vi "Create Song.vi"(0 "Name":string, 5 "Duration (s)":T1 format="%<%M:%S>T", 7 "Artist":string, 9 "Album":string, 11 "error in (no error)":errorcluster) -> (4 "Song out":refnum<class "Song.lvclass">, 15 "error out":errorcluster)   [LabVIEW 2015, in "Song.lvclass"]
uses:
  Song.lvclass
  Song Duration.ctl
  Song.lvclass/Song.ctl
  Write Duration (s).vi
  Write Artist.vi
  Write Album.vi
  MusicElement.lvclass
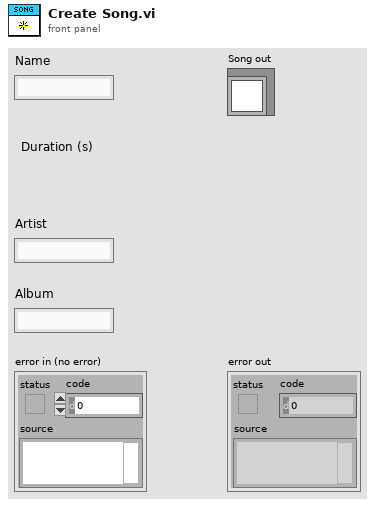
[diagram p1: front panel]
types:
  T1 = typedef "Song.lvclass/Song Duration.ctl" = timestamp
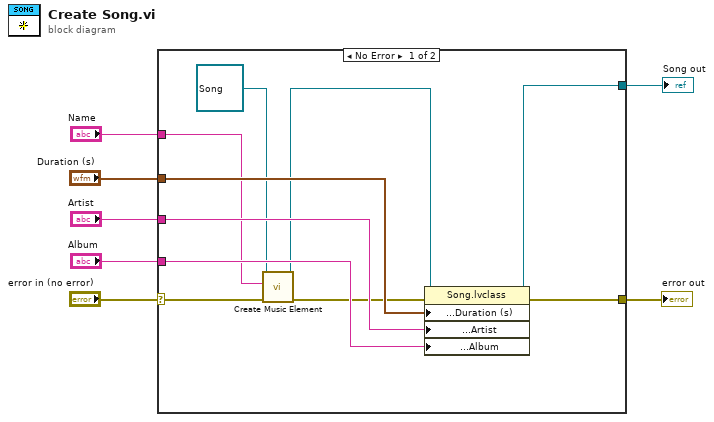
[diagram p0: block diagram]
diagram:
  n1 = case shown="No Error" "error in (no error)" {
    selector: "error in (no error)" -> [w12 w18]
    tunnel: [w16 w18] -> w6
    tunnel: "Name" -> [w8 _]
    tunnel: [w17 _] -> w4
    tunnel: "Artist" -> [w15 _]
    tunnel: "Album" -> [w14 _]
    tunnel: "Duration (s)" -> [w13 _]
    frame No Error {
      n2 = call "Create Music Element.vi"("error in (no error)"=w12, "Name"=w8, "MusicElement in"=refnum<class "Song.lvclass"> refnum ("Song out")) -> ("error out"=w9:errorcluster, "MusicElement out"=w10:refnum<class "Song.lvclass">)  [unwired: 7 in]
      n3 = property class="Song.lvclass"(reference=w10, error in=w9, "API:Data Member Accessors:Duration (s)"=w13, "API:Data Member Accessors:Artist"=w15, "API:Data Member Accessors:Album"=w14) -> (reference out=w17:refnum<class "Song.lvclass">, error out=w16:errorcluster)
    }
    frame Error {
    }
  }
  "error out" <- w6
  "Song out" <- w4
